vi "PH_PPPA_PowerUnit.panel.vi"() -> ()   [LabVIEW 2014, in "PH_PPPA_PowerUnit.lvlib"]
uses:
  PH_PPPA_PowerUnit.lvlib
  PH_PowerUnit_BaseClass/PH_PowerUnit_BaseClass.SM States.ctl
  PH_StatusHandler/PH_StatusHandler.GUI element.ctl
  PH_PowerUnit_BaseClass/PH_PowerUnit_BaseClass.GUI Refs to pack.ctl
  PH_PowerUnit_BaseClass/PH_PowerUnit_BaseClass.GUI Refs.ctl
  CSCore/CSObj/CSObj.lvlib
  PH_Common/PH_Common.lvlib
  PH_PowerUnit_BaseClass/PH_PowerUnit_BaseClass.lvlib
  PH_Class/PH_Class.lvlib
  PH_StatusHandler/PH_StatusHandler.lvlib
panel:
  out "Seq SM State":string
  out "PSDB Status":u32(colorbox)=6618880 caption="PSDB"
  out "Timing":u32(colorbox)=6618880
  out "Status":T1 caption="State PU"
  out "Timeout SM":T2 caption="State PU"
  out "State SM":T2 caption="State PU"
  out "Chiller":u32(colorbox)=9567230
  out "Trigger":u32(colorbox)
  out "PSU":u32(colorbox)
  out "EOC":u32(colorbox)
  out "Ignitron":u32(colorbox)=6618880
  in  "PU on":bool
  out "Rossrelais":u32(colorbox) caption="Dump RR"
  in  "Set Voltage":dbl
  in  "Exit":bool
  in  "Fire":bool
  out "Waiting Time":dbl=999999.0
  out "Water":u32(colorbox)
  out "Mercury":u32(colorbox)
  out "error out":errorcluster
  in  "Delete":bool
  in  "error in (no error)":errorcluster
  in  "object ref":refnum<vi>
  out "PreAmp":u32(colorbox)
  # "PCS"
  # "3.40"
  # "V"
  # "s"
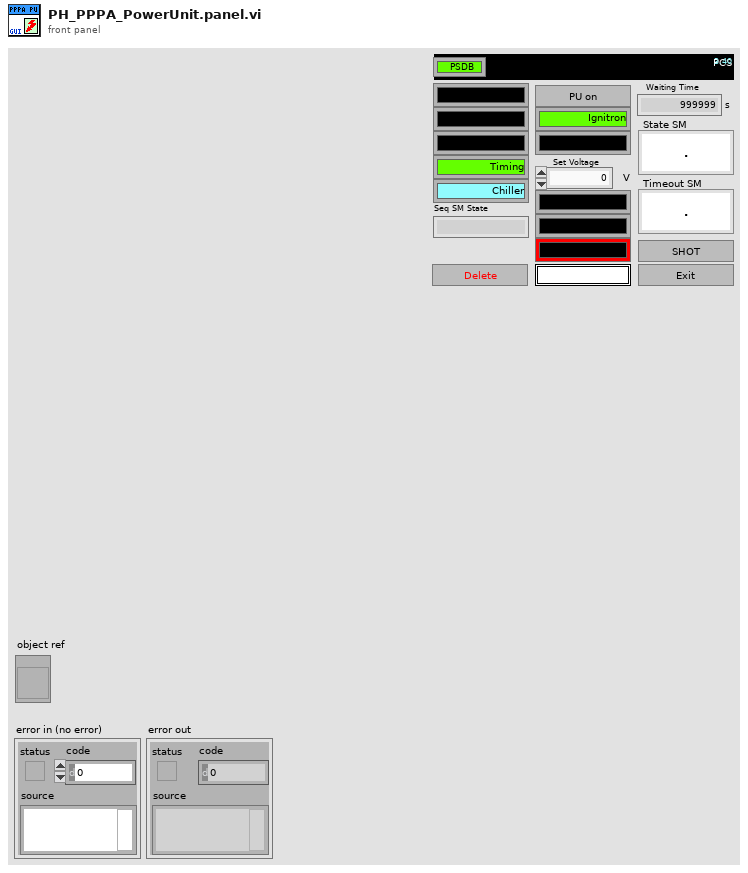
[diagram p1: front panel]
types:
  T1 = typedef "PH_StatusHandler.lvlib/PH_StatusHandler.GUI element.ctl" = u16
  T2 = typedef "PH_PowerUnit_BaseClass.lvlib/PH_PowerUnit_BaseClass.SM States.ctl" = enum16{".", "Stand by", "Switch PU on", "Configure", "Set Default Voltage", "Set STANDBY", "Set READY", "Wait for Shot Cmd", "Open Dump Rods", "Open Ross Relais", "Close Ross Relais", "Switch PSU on", "Switch PSU off", "Charge", "Switch GD Channel on", "Close Dump Rods", "Rods-TO", "RR-TO", "PSU-TO", "Trigger-TO"}
  T3 = typedef "PH_PowerUnit_BaseClass.lvlib/PH_PowerUnit_BaseClass.GUI Refs to pack.ctl" = cluster{"GUI Refs":T4, "Enabled":refnum<vi>, "PU on":refnum<vi>, "Waiting Time":refnum<vi>, "Timing.Instance":refnum<vi>, "Seq SM State":refnum<vi>, "Subscribed Trendmssgs":refnum<vi>[]}
  T4 = typedef "PH_PowerUnit_BaseClass.lvlib/PH_PowerUnit_BaseClass.GUI Refs.ctl" = cluster{"Delete Inst":refnum<vi>, "State TO SM":refnum<vi>, "State SM":refnum<vi>, "Fire":refnum<vi>}
  T5 = cluster{"GUI Refs Power Unit Base Class":T3, "PSDB Status":refnum<vi>}
  T6 = typedef "PH_PowerUnit_BaseClass.lvlib/PH_PowerUnit_BaseClass.i attribute.ctl" = cluster{"Constructor finished":bool, "PU":cluster{"In use":bool, "Service ID in use":i32, "GUI Ref":refnum<vi>}, "Enabling":cluster{"State":T7, "GUI Ref":refnum<vi>}, "Timing":cluster{"Last Shot":dbl, "Time between Shots [Sec]":dbl, "Waiting Time over?":bool, "Service ID Waiting Time":i32, "GUI Ref":refnum<vi>, "Instance":cluster{"Status":T8, "linked?":bool, "GUI Ref":refnum<vi>}}, "Sequencer":cluster{"SM State":string, "GUI Ref":refnum<vi>, "linked":bool}, "Subscribed Trendmssgs":cluster{"Tagname":string, "Status":T8, "linked?":bool, "Shot Condition":T8, "GUI Ref":refnum<vi>}[], "PP PU":T9, "Default Voltage (V)":dbl, "GUI Refs":T4, "PSDB data":cluster{"Shot Voltage [V]":dbl, "State TO SM":T2, "Write 2 early":bool}, "State TO SM":T2}
  T7 = typedef "PH_SystemInformation.lvlib/PH_SystemInformationEnabling State.ctl" = i32
  T8 = typedef "PH_StatusHandler.lvlib/PH_StatusHandler.Status.ctl" = i16
  T9 = typedef "PH_PP_Common.lvlib/PH_PP_Common.PUs.ctl" = enum16{"no Info", "PA-19mm-1", "PA-19mm-2", "PA-45mm-PILC", "PA-45mm-MAIN", "MA-PU-1", "MA-PU-2", "MA-PU-3", "MA-PU-4", "MA-PU-5", "MA-PU-6", "MA-FR", "MA-PILC", "PA-45mm-DP"}
  T10 = typedef "PH_PPPA_PowerUnit.lvlib/PH_PPPA_PowerUnit.i attribute.ctl" = cluster{"GUI Refs":cluster{"Ignitron":refnum<vi>, "Rossrelais":refnum<vi>, "Set Voltage":refnum<vi>, "PSU":refnum<vi>, "EOC":refnum<vi>, "Trigger":refnum<vi>}, "Ignitron":T11, "PSU":T12, "Dump Ross Relais":T13, "Trigger":cluster{"State Device":T8, "linked?":bool}, "Timing Settings":cluster{"Prdc Fast?":bool, "Default Value Periodic Interval":i32, "Mercury on since":dbl, "Warm up Time Mercury [s]":dbl}, "Set Voltage [V]":dbl, "19er Ignitionbox":string}
  T11 = typedef "PH_PP_Common.lvlib/PH_PP_Common.Ignitron Attributes.ctl" = cluster{"State Device":T8, "linked?":bool}
  T12 = typedef "PH_PP_Common.lvlib/PH_PP_Common.PSU Attributes.ctl" = cluster{"lower limit [V]":dbl, "upper limit [V]":dbl, "Voltage set":bool, "State Device":T8, "linked?":bool}
  T13 = typedef "PH_PP_Common.lvlib/PH_PP_Common.Ross Relais Attributes.ctl" = cluster{"State Device":T8, "linked?":bool}
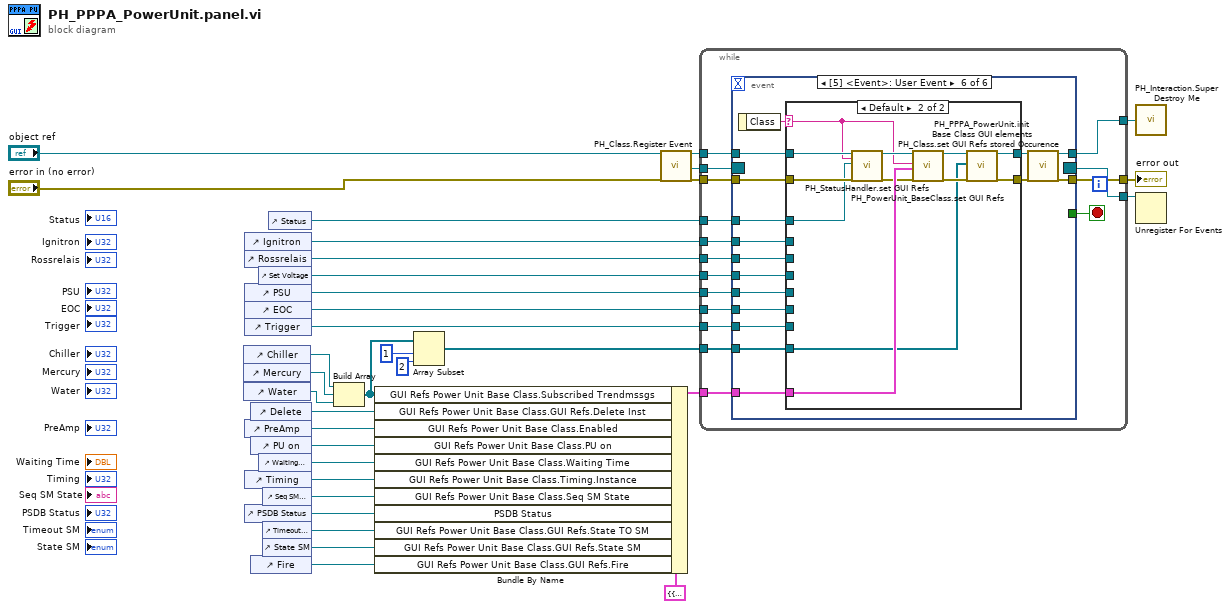
[diagram p0: block diagram]
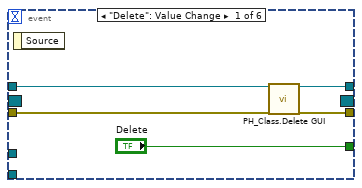
[diagram p2: hidden frame]
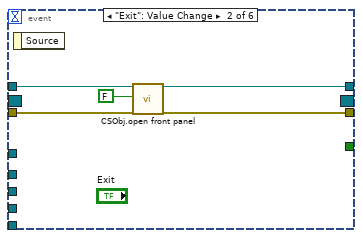
[diagram p3: hidden frame]
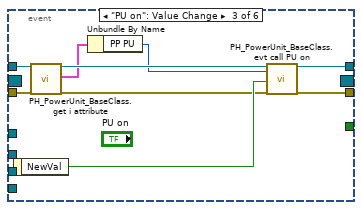
[diagram p4: hidden frame]
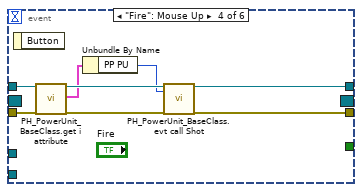
[diagram p5: hidden frame]
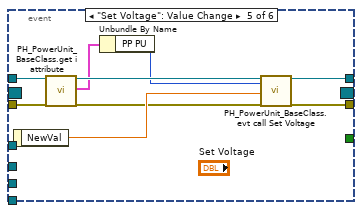
[diagram p6: hidden frame]
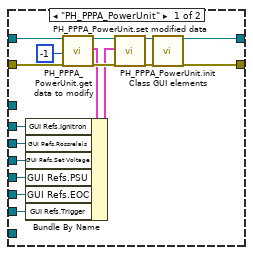
[diagram p7: hidden frame]
diagram:
  n1 = control-ref of="Chiller"() -> (w30:refnum<vi>)
  n2 = control-ref of="Mercury"() -> (w32:refnum<vi>)
  n3 = control-ref of="Water"() -> (w31:refnum<vi>)
  n4 = control-ref of="Ignitron"() -> (w11:refnum<vi>)
  n5 = control-ref of="Rossrelais"() -> (w12:refnum<vi>)
  n6 = control-ref of="PSU"() -> (w14:refnum<vi>)
  n7 = control-ref of="EOC"() -> (w15:refnum<vi>)
  n8 = control-ref of="Trigger"() -> (w16:refnum<vi>)
  n9 = control-ref of="PreAmp"() -> (w23:refnum<vi>)
  n10 = control-ref of="Timing"() -> (w20:refnum<vi>)
  n11 = control-ref of="PSDB Status"() -> (w18:refnum<vi>)
  n12 = control-ref of="Delete"() -> (w24:refnum<vi>)
  n13 = control-ref of="PU on"() -> (w22:refnum<vi>)
  n14 = control-ref of="Fire"() -> (w2:refnum<vi>)
  n15 = control-ref of="Set Voltage"() -> (w13:refnum<vi>)
  n16 = control-ref of="Waiting Time"() -> (w21:refnum<vi>)
  n17 = control-ref of="Seq SM State"() -> (w19:refnum<vi>)
  n18 = control-ref of="Timeout SM"() -> (w3:refnum<vi>)
  n19 = control-ref of="State SM"() -> (w4:refnum<vi>)
  n20 = control-ref of="Status"() -> (w1:refnum<vi>)
  n21 = Build Array(w30, w32, w31) -> (w7:refnum<vi>[])
  n22 = Bundle By Name(cluster=T5 {"GUI Refs Power Unit Base Class"={"GUI Refs"={"Delete Inst"=refnum, "State TO SM"=refnum, "State SM"=refnum, "Fire"=refnum}, "Enabled"=refnum, "PU on"=refnum, "Waiting Time"=refnum, "Timing.Instance"=refnum, "Seq SM State"=refnum, "Subscribed Trendmssgs"=[]}, "PSDB Status"=refnum} ("GUI Refs"), "GUI Refs Power Unit Base Class.Subscribed Trendmssgs"=w7, "GUI Refs Power Unit Base Class.GUI Refs.Delete Inst"=w24, "GUI Refs Power Unit Base Class.Enabled"=w23, "GUI Refs Power Unit Base Class.PU on"=w22, "GUI Refs Power Unit Base Class.Waiting Time"=w21, "GUI Refs Power Unit Base Class.Timing.Instance"=w20, "GUI Refs Power Unit Base Class.Seq SM State"=w19, "PSDB Status"=w18, "GUI Refs Power Unit Base Class.GUI Refs.State TO SM"=w3, "GUI Refs Power Unit Base Class.GUI Refs.State SM"=w4, "GUI Refs Power Unit Base Class.GUI Refs.Fire"=w2) -> (w17:T5)
  n23 = Array Subset(array=w7, index=1, length=2) -> (w5:refnum<vi>[])
  n24 = call "PH_Class.Register Event.vi"("i ref in"="object ref", "error in (no error)"="error in (no error)") -> ("i ref out"=w29:refnum<vi>, "Event Registration Refnum"=w27:refnum<event-registration>, "error out"=w28:errorcluster)  [unwired: 15 in]
  n25 = while {
    tunnel: w29 -> [w47]
    tunnel: [w46] -> w34
    tunnel: [w49] -> w33
    tunnel: w28 -> [w48]
    tunnel: w27 -> [w45]
    tunnel: [w44] -> w26
    tunnel: w17 -> [w43]
    tunnel: w16 -> [w42]
    tunnel: w15 -> [w41]
    tunnel: w14 -> [w40]
    tunnel: w13 -> [w39]
    tunnel: w12 -> [w38]
    tunnel: w11 -> [w37]
    tunnel: w5 -> [w36]
    tunnel: w1 -> [w35]
    stop <- w50 stop-if-true
    n26 = event shown="[5] <Event>: User Event" {
      selector: w45 -> [_ _ _ _ _ _]
      dyn-events: [_ _ _ _ _ _] -> w44
      timeout: _ -> [_ _ _ _ _ _]
      tunnel: ["Delete" _ _ _ _ _] -> w50
      tunnel: w47 -> [w52 w58 w64 w73 w81 w102]
      tunnel: [w53 w59 w68 w76 w85 w97] -> w49
      tunnel: w48 -> [w54 w60 w69 w77 w86 w101]
      tunnel: [w51 w56 w66 w75 w83 w98] -> w46
      tunnel: w43 -> [_ _ _ _ _ w95]
      tunnel: w42 -> [_ _ _ _ _ w94]
      tunnel: w41 -> [_ _ _ _ _ w93]
      tunnel: w40 -> [_ _ _ _ _ w92]
      tunnel: w39 -> [_ _ _ _ _ w91]
      tunnel: w38 -> [_ _ _ _ _ w90]
      tunnel: w37 -> [_ _ _ _ _ w89]
      tunnel: w36 -> [_ _ _ _ _ w88]
      tunnel: w35 -> [_ _ _ _ _ w87]
      event "Delete": Value Change {
        n27 = event-data() -> ()  [unwired: 1 in, 1 out]
        n28 = call "PH_Class.Delete GUI.vi"("VI in"=w52, "error in (no error)"=w54) -> ("VI out"=w51:refnum<vi>, "error out"=w53:errorcluster)  [unwired: 16 in]
      }
      event "Exit": Value Change {
        n29 = event-data() -> ()  [unwired: 1 in, 1 out]
        n30 = call "CSObj.open front panel.vi"("i ref in"=w58, "frontPanelOpen"=FALSE ("front panel open"), "error in (no error)"=w60) -> ("i ref out"=w56:refnum<vi>, "error out"=w59:errorcluster)  [unwired: 15 in]
      }
      event "PU on": Value Change {
        n31 = event-data() -> ("NewVal"=w67:bool)  [unwired: 1 in]
        n32 = call "PH_PowerUnit_BaseClass.get i attribute.vi"("i ref in"=w64, "error in (no error)"=w69) -> ("i ref out"=w63:refnum<vi>, "i attribute"=w62:T6, "error out"=w65:errorcluster)  [unwired: 15 in]
        n33 = Unbundle By Name(w62) -> ("PP PU"=w61:T9)
        n34 = call "PH_PowerUnit_BaseClass.evt call PU on.vi"("i ref in"=w63, "PowerUnit"=w61, "PU on"=w67, "error in (no error)"=w65) -> ("i ref out"=w66:refnum<vi>, "error out"=w68:errorcluster)  [unwired: 14 in]
      }
      event "Fire": Mouse Up {
        n35 = event-data() -> ()  [unwired: 1 in, 1 out]
        n36 = call "PH_PowerUnit_BaseClass.get i attribute.vi"("i ref in"=w73, "error in (no error)"=w77) -> ("i ref out"=w72:refnum<vi>, "i attribute"=w71:T6, "error out"=w74:errorcluster)  [unwired: 15 in]
        n37 = Unbundle By Name(w71) -> ("PP PU"=w70:T9)
        n38 = call "PH_PowerUnit_BaseClass.evt call Shot.vi"("i ref in"=w72, "PowerUnit"=w70, "error in (no error)"=w74) -> ("i ref out"=w75:refnum<vi>, "error out"=w76:errorcluster)  [unwired: 15 in]
      }
      event "Set Voltage": Value Change {
        n39 = event-data() -> ("NewVal"=w84:dbl)  [unwired: 1 in]
        n40 = call "PH_PowerUnit_BaseClass.get i attribute.vi"("i ref in"=w81, "error in (no error)"=w86) -> ("i ref out"=w80:refnum<vi>, "i attribute"=w79:T6, "error out"=w82:errorcluster)  [unwired: 15 in]
        n41 = Unbundle By Name(w79) -> ("PP PU"=w78:T9)
        n42 = call "PH_PowerUnit_BaseClass.evt call Set Voltage.vi"("i ref in"=w80, "PowerUnit"=w78, "Voltage [V]"=w84, "error in (no error)"=w82) -> ("i ref out"=w83:refnum<vi>, "error out"=w85:errorcluster)  [unwired: 14 in]
      }
      event User Event {
        n43 = event-data() -> ("Class"=w96:string)  [unwired: 1 in]
        n44 = case shown="Default" w96 {
          selector: w96 -> [_ w121]
          tunnel: w102 -> [w114 w123]
          tunnel: w101 -> [w113 w131]
          tunnel: [w103 w126] -> w100
          tunnel: [w104 w128] -> w99
          tunnel: w95 -> [_ w130]
          tunnel: w94 -> [w111 _]
          tunnel: w93 -> [w110 _]
          tunnel: w92 -> [w109 _]
          tunnel: w91 -> [w108 _]
          tunnel: w90 -> [w107 _]
          tunnel: w89 -> [w106 _]
          tunnel: w88 -> [_ w125]
          tunnel: w87 -> [_ w120]
          frame "PH_PPPA_PowerUnit" {
            n45 = call "PH_PPPA_PowerUnit.get data to modify.vi"("i ref in"=w114, "ms timeout (10000)"=-1, "error in (no error)"=w113) -> ("i ref out"=w117:refnum<vi>, "i attribute"=w116:T10, "error out"=w119:errorcluster)  [unwired: 13 in, 1 out]
            n46 = Bundle By Name(cluster=w116, "GUI Refs.Ignitron"=w106, "GUI Refs.Rossrelais"=w107, "GUI Refs.Set Voltage"=w108, "GUI Refs.PSU"=w109, "GUI Refs.EOC"=w110, "GUI Refs.Trigger"=w111) -> (w115:T10)
            n47 = call "PH_PPPA_PowerUnit.set modified data.vi"("i ref in"=w117, "i attribute"=w115, "error in (no error)"=w119) -> ("i ref out"=w105:refnum<vi>, "error out"=w112:errorcluster)  [unwired: 15 in]
            n48 = call "PH_PPPA_PowerUnit.init Class GUI elements.vi"("VI in"=w105, "error in (no error)"=w112) -> ("VI out"=w104:refnum<vi>, "error out"=w103:errorcluster)  [unwired: 16 in]
          }
          frame Default {
            n49 = call "PH_StatusHandler.set GUI Refs.vi"("i ref in"=w123, "Class"=w121, "GUI Ref"=w120, "error in (no error)"=w131) -> ("i ref out"=w122:refnum<vi>, "error out"=w124:errorcluster)  [unwired: 14 in]
            n50 = call "PH_PowerUnit_BaseClass.set GUI Refs.vi"("i ref  in"=w122, "Class"=w121, "GUI Refs"=w130, "error in"=w124) -> ("i ref out"=w129:refnum<vi>, "error out"=w127:errorcluster)  [unwired: 14 in]
            n51 = call "PH_PPPA_PowerUnit.init Base Class GUI elements.vi"("VI in"=w129, "GUI Refs Array to be set unvisible"=w125, "error in (no error)"=w127) -> ("VI out"=w128:refnum<vi>, "error out"=w126:errorcluster)  [unwired: 15 in]
          }
        }
        n52 = call "PH_Class.set GUI Refs stored Occurence.vi"("i ref in"=w99, "error in (no error)"=w100) -> ("i ref out"=w98:refnum<vi>, "error out"=w97:errorcluster)  [unwired: 16 in]
      }
    }
  }
  "error out" <- w33
  n53 = call "PH_Interaction.Super Destroy Me.vi"("i ref out"=w34) -> ()
  n54 = Unregister For Events(event registration refnum=w26) -> ()  [unwired: 1 in, 1 out]
